vi "ENPH 354 Assignment 1 - Q8.vi"() -> ()   [LabVIEW 2021]
panel:
  out "Numeric":dbl
  out "Array 2":dbl[](array[numeric])
  in  "Array":bool[](array[boolean])
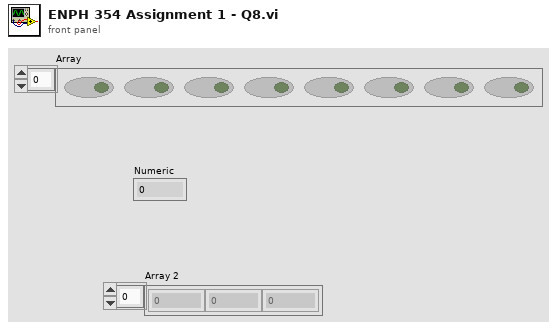
[diagram p1: front panel]
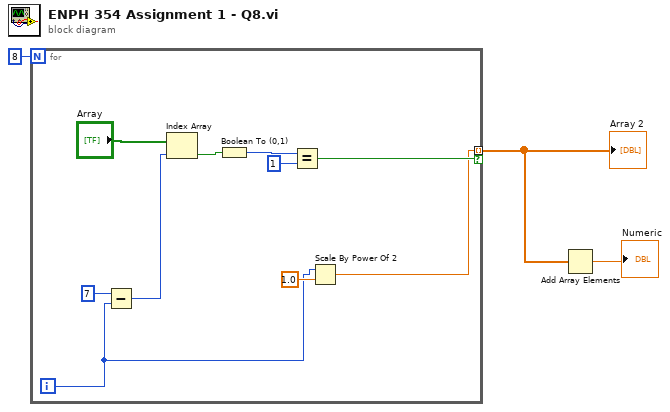
[diagram p0: block diagram]
diagram:
  n1 = for {
    N: 8 -> [_]
    tunnel: [w5] -> w2 mode=indexing if=w7
    i -> [w4]
    n2 = Subtract(x=7, y=w4) -> (x-y=w11:i32)
    n3 = Index Array(array="Array", index=w11) -> (element=w10:bool)
    n4 = Boolean To (0,1)(Boolean=w10) -> (0, 1=w9:i16)
    n5 = Equal?(x=w9, y=i16 1) -> (x = y?=w7:bool)
    n6 = Scale By Power Of 2(n=w4, x=1.0) -> (x*2^n=w5:dbl)
  }
  "Array 2" <- w2
  n7 = Add Array Elements(numeric array=w2) -> (sum=→"Numeric":dbl)
